vi "Connect.vi"(8 "error in":errorcluster, 11 "ManualPS in":refnum<class "ManualPS.lvclass">) -> (0 "error out":errorcluster, 3 "ManualPS out":refnum<class "ManualPS.lvclass">)   [LabVIEW 2018, in "ManualPS.lvlib" / "ManualPS.lvclass"]
uses:
  ManualPS.lvclass
panel:
  in  "OK Button":bool
  # "Verify power supply is turned on"
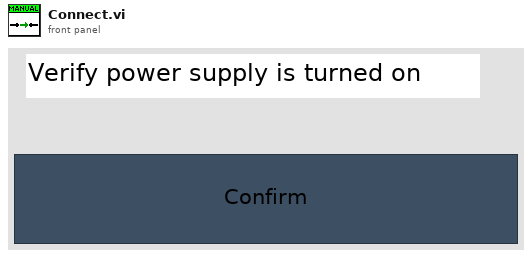
[diagram p1: front panel]
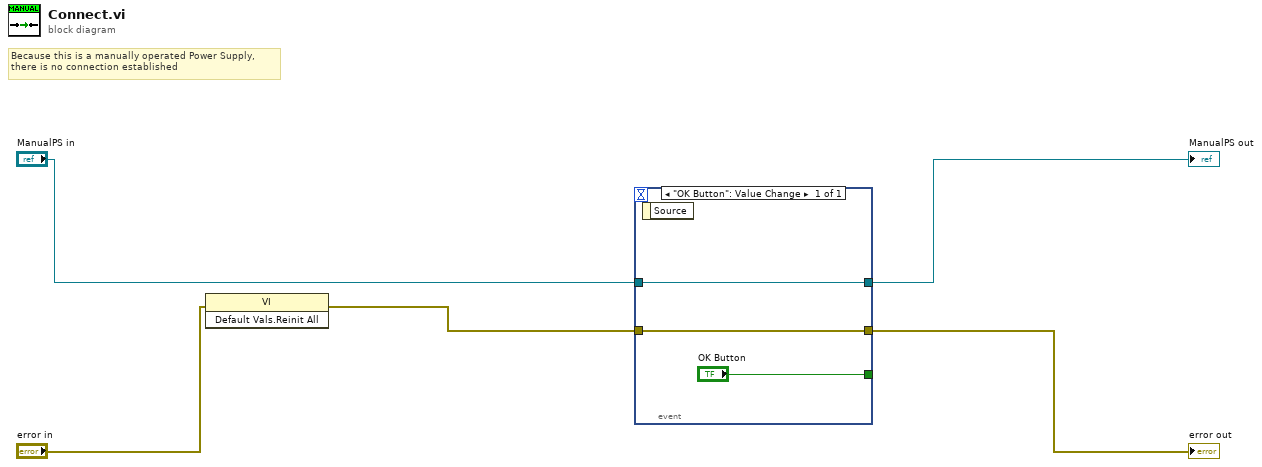
[diagram p0: block diagram]
diagram:
  # "Because this is a manually operated Power Supply, \nthere is no connection established"
  n1 = invoke class="VI" method="Default Vals.Reinit All"(error in="error in") -> (error out=w1:errorcluster)  [unwired: 2 in, 2 out]
  n2 = event shown="[0] \"OK Button\": Value Change" {
    selector: _ -> [_]
    dyn-events: _ -> [_]
    timeout: _ -> [_]
    tunnel: "ManualPS in" -> [w7]
    tunnel: w1 -> [w8]
    tunnel: [w8] -> w4
    tunnel: [w7] -> w3
    tunnel: ["OK Button"] -> _
    event "OK Button": Value Change {
      n3 = event-data() -> ()  [unwired: 1 in, 1 out]
    }
  }
  "error out" <- w4
  "ManualPS out" <- w3
